vi "Fluence in Tile.vi"(0 "Analyze Fluence in":refnum<class "Analyze Fluence.lvclass">, 5 "Image in":T1, 11 "error in (no error)":errorcluster) -> (4 "Analyze Fluence out":refnum<class "Analyze Fluence.lvclass">, 6 "Image Dst Out":T1, 8 "Max Fluence":dbl[unit], 10 "fluence infos":T2[](array[typedef]), 15 "error out":errorcluster)   [LabVIEW 2014, in "Analyze.lvlib" / "Analyze Fluence.lvclass"]
uses:
  Analyze Fluence.lvclass
  Fluence Info.ctl
  <vilib>/vision/Image Controls.llb/IMAQ Image.ctl
  Analyze Parameter/Analyze Parameter Fluence/Analyze Parameter Fluence.lvclass
  Analyze Parameter/Analyze Parameter Energy/Analyze Parameter Energy.lvclass
  Analyze Fluence.lvclass/Analyze Fluence.ctl
  Analyze Parameter/Analyze Parameter Energy/Analyze Parameter Energy.lvclass/Analyze Parameter Energy.ctl
  <vilib>/vision/NI_Vision_Development_Module.lvlib
  Analyze BaseClass/Analyze BaseClass/Analyze BaseClass.lvclass
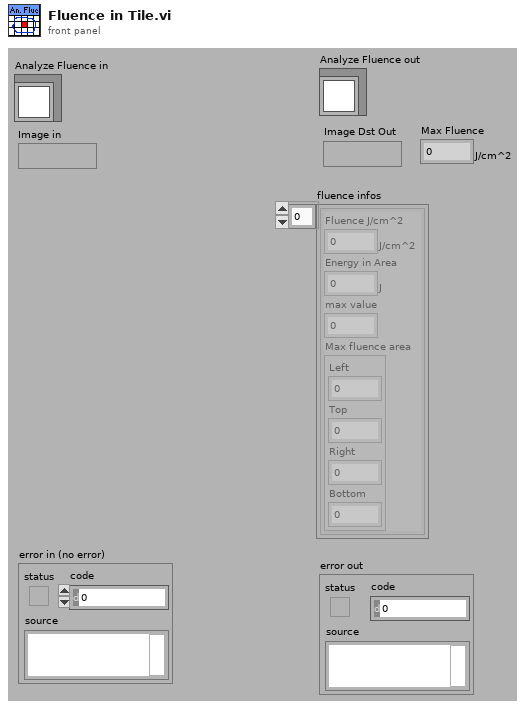
[diagram p1: front panel]
types:
  T1 = typedef "IMAQ Image.ctl" = refnum<image>
  T2 = typedef "Analyze.lvlib/Analyze Fluence.lvclass/Fluence Info.ctl" = cluster{"Fluence J/cm^2":dbl[unit], "Energy in Area":dbl[unit], "max value":i64, "Max fluence area":cluster{"Left":i32, "Top":i32, "Right":i32, "Bottom":i32}}
  T3 = cluster{"Left":i32, "Top":i32, "Right":i32, "Bottom":i32}
  T4 = typedef "Image Type" = u32
  T5 = typedef "ROI Descriptor" = cluster{"Global Rectangle":i32[], "Contours":cluster{"ID":enum32{"External", "Internal"}, "Type":u32, "Coordinates":i32[]}[]}
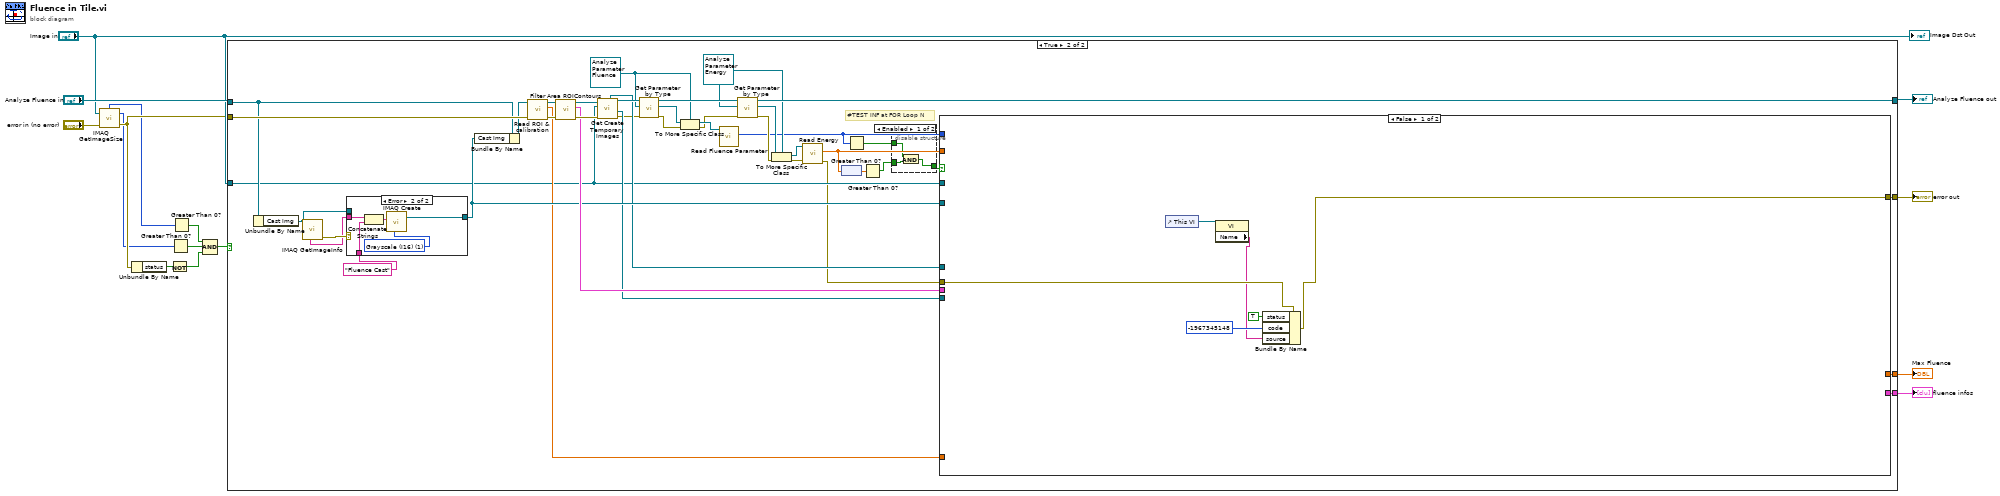
[diagram p0: block diagram]
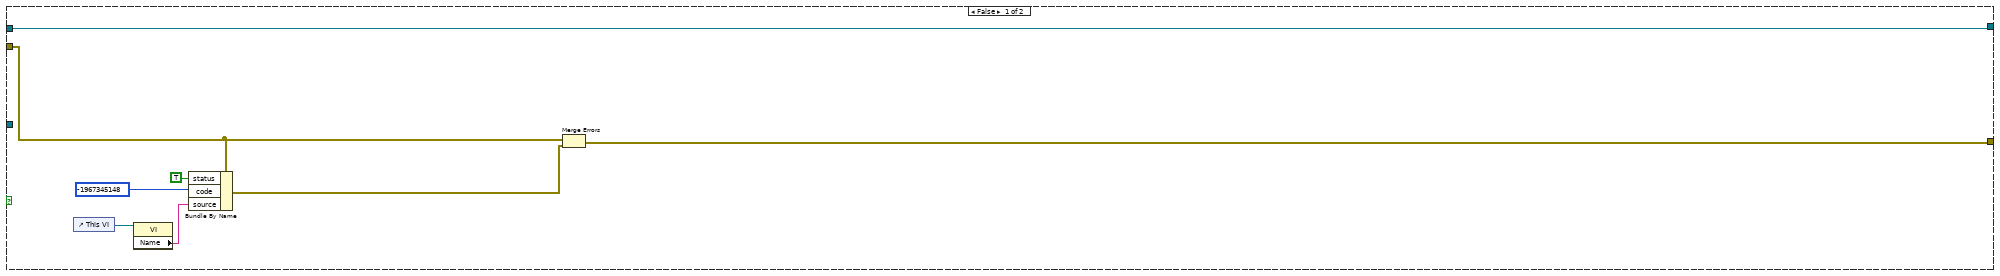
[diagram p2: hidden frame]
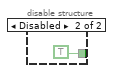
[diagram p3: hidden frame]
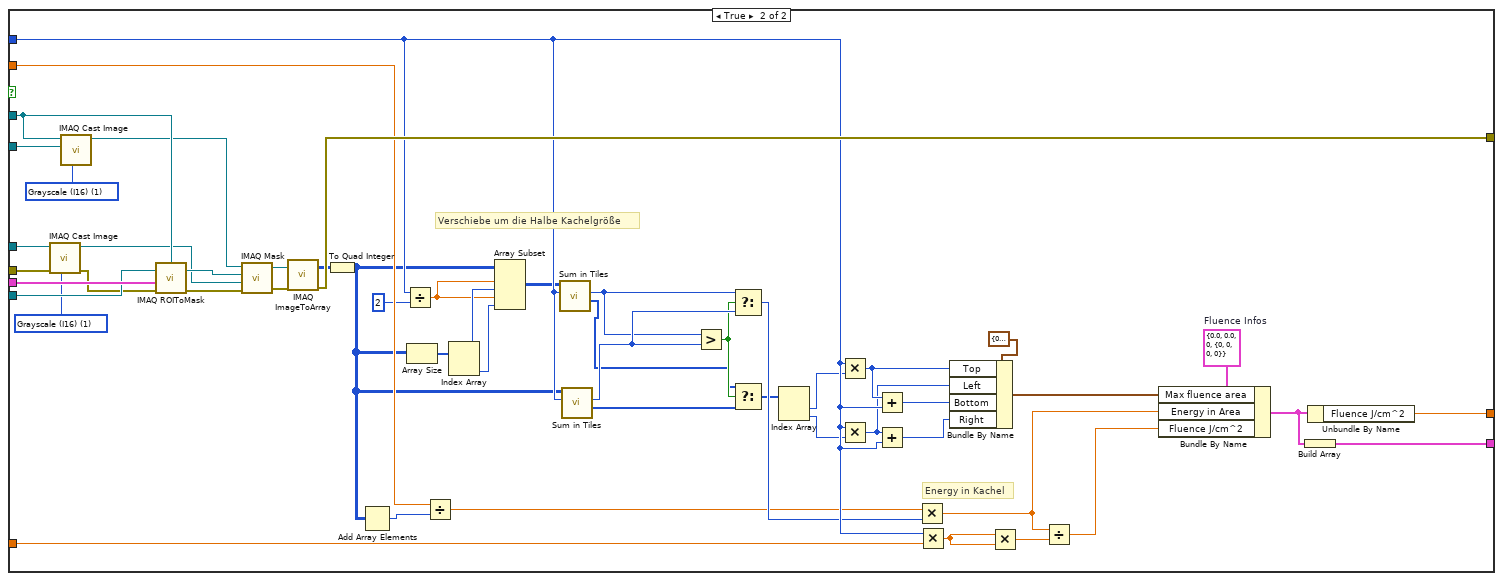
[diagram p4: hidden frame]
diagram:
  n1 = call "IMAQ GetImageSize"("Image"="Image in", "error in (no error)"="error in (no error)") -> ("Y Resolution"=w5:i32, "X Resolution"=w6:i32, "error out"=w8:errorcluster)  [unwired: 2 in]
  n2 = Unbundle By Name(w8) -> ("status"=w7:bool)
  n3 = Not(x=w7) -> (.not. x?=w2:bool)
  n4 = Greater Than 0?(x=w5) -> (x > 0?=w3:bool)
  n5 = Greater Than 0?(x=w6) -> (x > 0?=w4:bool)
  n6 = Compound Arithmetic op=AND(w4, w3, w2) -> (w1:bool)
  n7 = case shown="True" w1 {
    tunnel: [_ w64] -> w15
    tunnel: w8 -> [w16 w60]
    tunnel: "Analyze Fluence in" -> [w23 w56]
    tunnel: [w18 w46] -> w13
    tunnel: "Image in" -> [_ w45]
    tunnel: [_ w44] -> w12
    tunnel: [w23 w42] -> w11
    frame False {
      n8 = control-ref of="This VI"() -> (w22:refnum<vi>)
      n9 = property class="VI"(reference=w22) -> ("Name"=w21:string)  [unwired: 1 in, 2 out]
      n10 = Bundle By Name(cluster=w16, "status"=TRUE, "code"=-1967345148 ("error code (no error:0)"), "source"=w21) -> (w17:errorcluster)
      n11 = Merge Errors(w16, w17) -> (w18:errorcluster)
    }
    frame True {
      w36 = refnum<class "Analyze Parameter Energy.lvclass"> refnum ("Energy")
      w39 = refnum<class "Analyze Parameter Fluence.lvclass"> refnum ("Parameter")
      # "#TEST INF at FOR Loop N"
      n12 = Unbundle By Name(w56) -> ("Cast Img"=w52:T1)
      n13 = call "IMAQ GetImageInfo"("Image"=w52) -> ("error out"=w55:errorcluster, "Image Name"=w54:string)  [unwired: 3 in, 6 out]
      n14 = case shown="Error" w55 {
        tunnel: w54 -> [_ w131]
        tunnel: "Fluence Cast" -> [_ w129]
        tunnel: [w127 w128] -> w50
        tunnel: w52 -> [w127 _]
        frame No Error {
        }
        frame Error {
          w132 = T4 1 items=["Grayscale (U8)", "Grayscale (I16)", "Grayscale (SGL)", "Complex (CSG)", "RGB (U32)", "HSL (U32)", "RGB (U64)", "Grayscale (U16)"] ("Image Type")
          n15 = Concatenate Strings(w131, w129) -> (w130:string)
          n16 = call "IMAQ Create"("Image Name"=w130, "Image Type"=w132) -> ("New Image"=w128:T1)  [unwired: 3 in, 1 out]
        }
      }
      n17 = Bundle By Name(cluster=w56, "Cast Img"=w50) -> (w51:refnum<class "Analyze Fluence.lvclass">)
      n18 = call-dynamic "Read ROI & calibration.vi"("error in (no error)"=w60, "Analyze BaseClass in"=w51) -> ("error out"=w59:errorcluster, "calibration mm/px"=w48:dbl[unit], "Analyze BaseClass out"=w62:refnum<class "Analyze Fluence.lvclass">)  [unwired: 6 in, 1 out]
      n19 = call-dynamic "Filter Area ROIContours.vi"("error in (no error)"=w59, "Analyze BaseClass in"=w62) -> ("error out"=w58:errorcluster, "ROI of Area type"=w57:T5, "Analyze BaseClass out"=w61:refnum<class "Analyze Fluence.lvclass">)  [unwired: 7 in]
      n20 = call-dynamic "Get Create Temporary Images.vi"("error in (no error)"=w58, "Image in"=w45, "Analyze BaseClass in"=w61) -> ("error out"=w31:errorcluster, "image mask"=w47:T1, "Analyze BaseClass out"=w63:refnum<class "Analyze Fluence.lvclass">, "masked image"=w49:T1)  [unwired: 4 in, 1 out]
      n21 = call "Get Parameter by Type.vi"("error in (no error)"=w31, "Parameter Type"=w39, "Analyze BaseClass in"=w63) -> ("error out"=w35:errorcluster, "Parameter"=w41:refnum<class "Analyze Parameter Base.lvclass">, "Analyze BaseClass out"=w43:refnum<class "Analyze Fluence.lvclass">)  [unwired: 5 in, 1 out]
      n22 = To More Specific Class(target class=w39, reference=w41, error in=w35) -> (specific class reference=w40:refnum<class "Analyze Parameter Fluence.lvclass">, error out=w34:errorcluster)
      n23 = call "Read Fluence Parameter.vi"("Analyze Parameter Fluence in"=w40) -> ("Size of region (px)"=w29:i32)  [unwired: 7 in, 3 out]
      n24 = call "Get Parameter by Type.vi"("error in (no error)"=w34, "Parameter Type"=w36, "Analyze BaseClass in"=w43) -> ("error out"=w33:errorcluster, "Parameter"=w37:refnum<class "Analyze Parameter Base.lvclass">, "Analyze BaseClass out"=w42:refnum<class "Analyze Fluence.lvclass">)  [unwired: 5 in, 1 out]
      n25 = To More Specific Class(target class=w36, reference=w37, error in=w33) -> (specific class reference=w38:refnum<class "Analyze Parameter Energy.lvclass">, error out=w32:errorcluster)
      n26 = call "Read Energy.vi"("error in (no error)"=w32, "Analyze Parameter Energy in"=w38) -> ("error out"=w30:errorcluster, "Energy"=w28:dbl[unit])  [unwired: 7 in, 1 out]
      n27 = node(w28) -> (w27:dbl)
      n28 = Greater Than 0?(x=w29) -> (x > 0?=w26:bool)
      n29 = Greater Than 0?(x=w27) -> (x > 0?=w25:bool)
      n30 = disable-structure shown="Enabled" {
        disable-tunnel: w26 -> [w67 _]
        disable-tunnel: w25 -> [w66 _]
        disable-tunnel: [w65 TRUE] -> w24
        frame Enabled {
          n31 = And(x=w67, y=w66) -> (x .and. y?=w65:bool)
        }
        frame Disabled {
        }
      }
      n32 = case shown="False" w24 {
        tunnel: [_ w126] -> w64
        tunnel: w57 -> [_ w125]
        tunnel: w50 -> [_ w124]
        tunnel: w49 -> [_ w123]
        tunnel: w48 -> [_ w122]
        tunnel: w47 -> [_ w121]
        tunnel: [w72 w120] -> w46
        tunnel: w45 -> [_ w119]
        tunnel: [_ w118] -> w44
        tunnel: w29 -> [_ w117]
        tunnel: w28 -> [_ w116]
        tunnel: w30 -> [w73 w115]
        frame False {
          n33 = control-ref of="This VI"() -> (w74:refnum<vi>)
          n34 = property class="VI"(reference=w74) -> ("Name"=w69:string)  [unwired: 1 in, 2 out]
          n35 = Bundle By Name(cluster=w73, "status"=TRUE, "code"=-1967345148 ("error code (no error:0)"), "source"=w69) -> (w72:errorcluster)
        }
        frame True {
          w80 = T2 {"Fluence J/cm^2"=0.0, "Energy in Area"=0.0, "max value"=0, "Max fluence area"={"Left"=0, "Top"=0, "Right"=0, "Bottom"=0}}  # Fluence Infos
          w107 = T4 1 items=["Grayscale (U8)", "Grayscale (I16)", "Grayscale (SGL)", "Complex (CSG)", "RGB (U32)", "HSL (U32)", "RGB (U64)", "Grayscale (U16)"] ("Image Type")
          w109 = T4 1 items=["Grayscale (U8)", "Grayscale (I16)", "Grayscale (SGL)", "Complex (CSG)", "RGB (U32)", "HSL (U32)", "RGB (U64)", "Grayscale (U16)"] ("Image Type")
          # "Verschiebe um die Halbe Kachelgröße"
          # "Energy in Kachel"
          n36 = call "IMAQ Cast Image"("Image Type"=w107, "error in (no error)"=w115, "Image Src"=w123) -> ("error out"=w106:errorcluster, "Image Dst Out"=w108:T1)  [unwired: 7 in]
          n37 = call "IMAQ Cast Image"("Image Type"=w109, "Image Dst"=w124, "Image Src"=w119) -> ("Image Dst Out"=w110:T1)  [unwired: 7 in, 1 out]
          n38 = call "IMAQ ROIToMask"("error in (no error)"=w106, "ROI Descriptor"=w125, "Image"=w121, "Image Model"=w119) -> ("error out"=w113:errorcluster, "Image Out"=w114:T1)  [unwired: 2 in, 1 out]
          n39 = call "IMAQ Mask"("error in (no error)"=w113, "Image Dst"=w108, "Image Mask"=w114, "Image Src"=w110) -> ("error out"=w92:errorcluster, "Image Dst Out"=w93:T1)  [unwired: 1 in]
          n40 = call "IMAQ ImageToArray"("error in (no error)"=w92, "Image"=w93) -> ("error out"=w120:errorcluster, "Image Pixels (I16)"=w112:i16[][])  [unwired: 2 in, 3 out]
          n41 = To Quad Integer(1:w112) -> (0:w111:i64[][])
          n42 = Add Array Elements(numeric array=w111) -> (sum=w105:i64)
          n43 = Divide(x=w117, y=2 ("x")) -> (x/y=w98:dbl)
          n44 = Array Size(array=w111) -> (size(s)=w99:i32[])
          n45 = Divide(x=w116, y=w105) -> (x/y=w95:dbl[unit])
          n46 = Index Array(array=w99) -> (element #1=w100:i32, element #2=w101:i32)  [unwired: 2 in]
          n47 = Array Subset(array=w111, index (row)=w98, length (row)=w100, index (col)=w98, length (col)=w101) -> (w102:i64[][])
          n48 = call "Sum in Tiles.vi"("size"=w117, "Image"=w102) -> ("Max Index"=w89:i32[], "Maximum"=w103:i64)  [unwired: 7 in, 1 out]
          n49 = call "Sum in Tiles.vi"("size"=w117, "Image"=w111) -> ("Max Index"=w88:i32[], "Maximum"=w104:i64)  [unwired: 7 in, 1 out]
          n50 = Greater?(x=w103, y=w104) -> (0:w90:bool)
          n51 = Select(t=w103, s=w90, f=w104) -> (s? t:f=w96:i64)
          n52 = Select(t=w89, s=w90, f=w88) -> (s? t:f=w87:i32[])
          n53 = Index Array(array=w87) -> (element #1=w86:i32, element #2=w85:i32)  [unwired: 2 in]
          n54 = Multiply(x=w117, y=w86) -> (x*y=w82:i32)
          n55 = Multiply(x=w117, y=w85) -> (x*y=w81:i32)
          n56 = Add(x=w82, y=w117) -> (x+y=w83:i32)
          n57 = Add(x=w81, y=w117) -> (x+y=w84:i32)
          n58 = Multiply(x=w95, y=w96) -> (x*y=w78:dbl[unit])
          n59 = Multiply(x=w117, y=w122) -> (x*y=w75:dbl[unit])
          n60 = Bundle By Name(cluster=T3 {"Left"=0, "Top"=0, "Right"=0, "Bottom"=0} ("Rectangle"), "Top"=w82, "Left"=w81, "Bottom"=w83, "Right"=w84) -> (w79:T3)
          n61 = Multiply(x=w75, y=w75) -> (x*y=w94:dbl[unit])
          n62 = Divide(x=w78, y=w94) -> (x/y=w77:dbl[unit])
          n63 = Bundle By Name(cluster=w80, "Max fluence area"=w79, "Energy in Area"=w78, "Fluence J/cm^2"=w77) -> (w76:T2)
          n64 = Build Array(w76) -> (w118:T2[])
          n65 = Unbundle By Name(w76) -> ("Fluence J/cm^2"=w126:dbl[unit])
        }
      }
    }
  }
  "fluence infos" <- w12
  "error out" <- w13
  "Max Fluence" <- w15
  "Analyze Fluence out" <- w11
  "Image Dst Out" <- "Image in"
